vi "Set State Message.vi"(6 "Configuration.State Message":bool, 8 "error in (no error)":errorcluster, 11 "Application Log in":refnum<class "Application Log.lvclass">) -> (0 "error out":errorcluster, 3 "Application Log out":refnum<class "Application Log.lvclass">)   [LabVIEW 2016, in "Stream Log.lvlib" / "Application Log.lvclass"]
doc: "--\nCopyright © 2017 Composed SystemsI All rights reserved.\n\nAuthor: Jon McBee <jon.mcbee@composed.io>\n\nThis library is provided \"AS IS\" ,WITHOUT WARRANTIES OR\nCONDITIONS OF ANY KIND, either express or implied.\n\nComposed Systems -- composed.io\n\nStream 0.0.1.1\nJon McBee - Composed Systems\nCopyright (c) 2017, Composed Systems"
uses:
  <userlib>/Composed Systems/Stream/Log/Application Log/Application Log.lvclass
  <userlib>/Composed Systems/Stream/Log/Application Log/Application Log.lvclass/Application Log.ctl
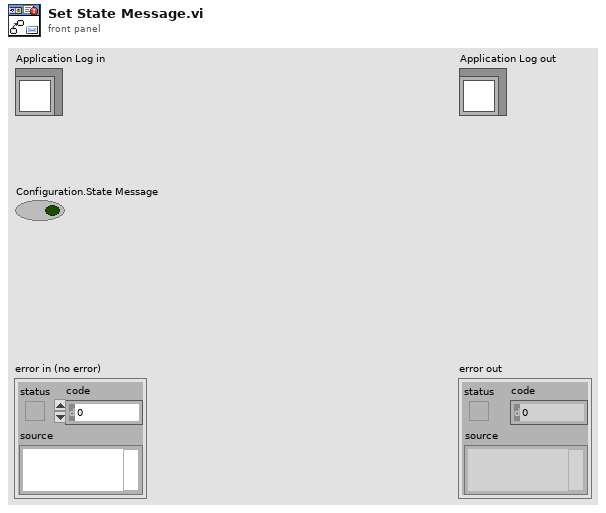
[diagram p1: front panel]
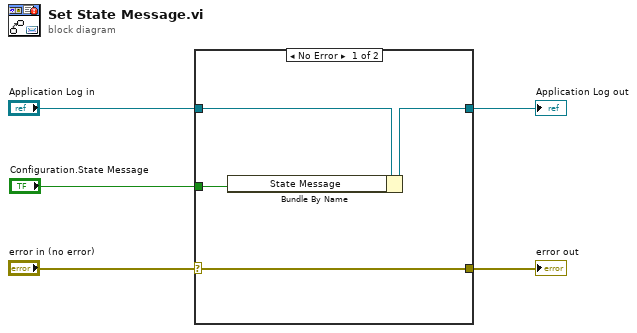
[diagram p0: block diagram]
diagram:
  n1 = case shown="No Error" "error in (no error)" {
    selector: "error in (no error)" -> [w9 w11]
    tunnel: [w9 w11] -> w4
    tunnel: [w7 w10] -> w2
    tunnel: "Application Log in" -> [w8 w10]
    tunnel: "Configuration.State Message" -> [w6 _]
    frame No Error {
      n2 = Bundle By Name(cluster=w8, "State Message"=w6) -> (w7:refnum<class "Application Log.lvclass">)
    }
    frame Error {
    }
  }
  "error out" <- w4
  "Application Log out" <- w2
